vi "SetColumnWidths.vi"(8 "error in (no error)":errorcluster, 11 "AdjustableMulticolumnListbox in":refnum<class "AdjMCLB.lvclass">) -> (0 "error out":errorcluster, 3 "AdjustableMulticolumnListbox out":refnum<class "AdjMCLB.lvclass">)   [LabVIEW 2020, in "AdjMCLB.lvclass"]
uses:
  AdjMCLB.lvclass
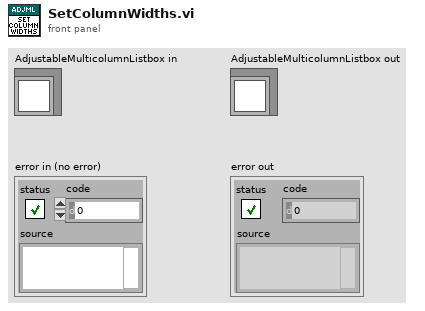
[diagram p1: front panel]
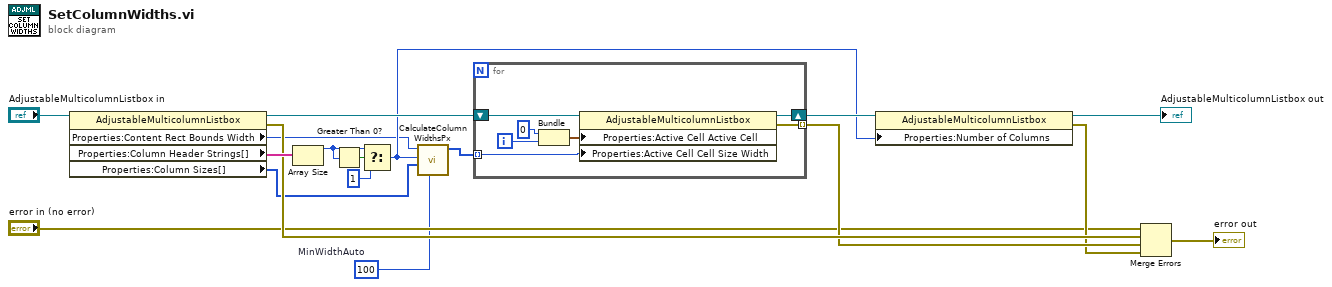
[diagram p0: block diagram]
diagram:
  w3 = 100  # MinWidthAuto
  n1 = property class="AdjustableMulticolumnListbox"(reference="AdjustableMulticolumnListbox in") -> (reference out=w13:refnum<class "AdjMCLB.lvclass">, error out=w10:errorcluster, "Properties:Content Rect Bounds Width"=w1:i32, "Properties:Column Header Strings[]"=w18:string[], "Properties:Column Sizes[]"=w5:i32[])  [unwired: 1 in]
  n2 = Array Size(array=w18) -> (size(s)=w14:i32)
  n3 = Greater Than 0?(x=w14) -> (x > 0?=w17:bool)
  n4 = Select(t=w14, s=w17, f=1) -> (s? t:f=w2:i32)
  n5 = call "CalculateColumnWidthsPx.vi"("MinWidthAuto"=w3, "Column Sizes[]"=w5, "NumberOfColumns"=w2, "ContentWidth"=w1) -> ("ColumnWidths (px)"=w4:i32[])  [unwired: 7 in]
  n6 = for {
    shift-right: [w24] -> w15
    shift-left: w13 -> [w25]
    tunnel: [w20] -> w9 mode=indexing
    tunnel: w4 -> [w19] mode=indexing
    i -> [w22]
    n7 = Bundle(0, w22) -> (w23:cluster{i32, i32})  [unwired: 1 in]
    n8 = property class="AdjustableMulticolumnListbox"(reference=w25, "Properties:Active Cell Active Cell"=w23, "Properties:Active Cell Cell Size Width"=w19) -> (reference out=w24:refnum<class "AdjMCLB.lvclass">, error out=w20:errorcluster)  [unwired: 1 in]
  }
  n9 = property class="AdjustableMulticolumnListbox"(reference=w15, "Properties:Number of Columns"=w2) -> (reference out=→"AdjustableMulticolumnListbox out":refnum<class "AdjMCLB.lvclass">, error out=w8:errorcluster)  [unwired: 1 in]
  n10 = Merge Errors("error in (no error)", w10, w9, w8) -> (→"error out":errorcluster)
